vi "Detect Stage Transitions.vi"(1 "Inj Event Boolean State Data":T1) -> (0 "Inj Event Boolean State Data out":T1)   [LabVIEW 2015]
uses:
  Types/Injection Capture Core Boolean State Data.ctl
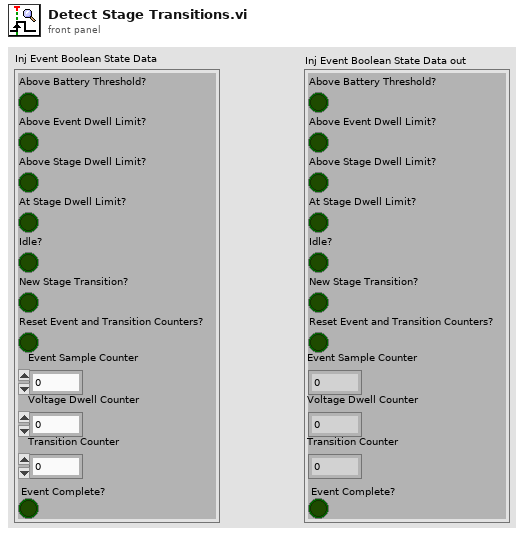
[diagram p1: front panel]
types:
  T1 = typedef "Injection Capture Core Boolean State Data.ctl" = cluster{"Above Battery Threshold?":bool, "Above Event Dwell Limit?":bool, "Above Stage Dwell Limit?":bool, "At Stage Dwell Limit?":bool, "Idle?":bool, "New Stage Transition?":bool, "Reset Event and Transition Counters?":bool, "Event Sample Counter":u16, "Voltage Dwell Counter":u32, "Transition Counter":u8, "Event Complete?":bool}
  T2 = enum8{"Wait for Start", "Wait for Pull-in", "Wait for End"}
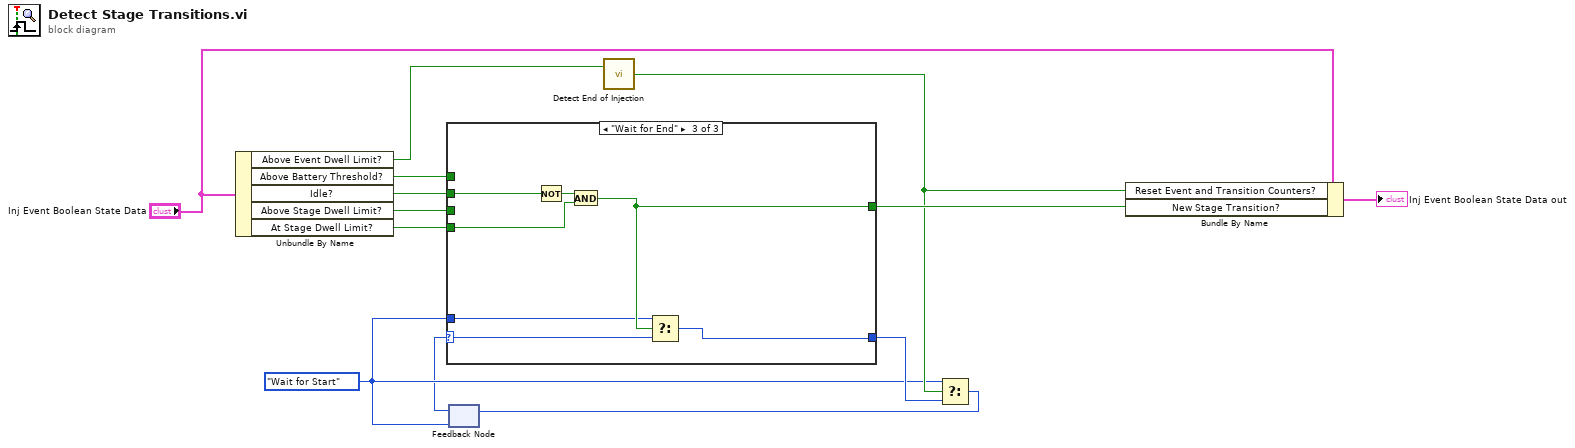
[diagram p0: block diagram]
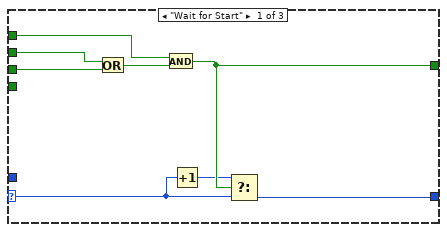
[diagram p2: hidden frame]
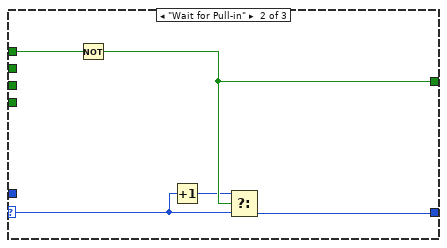
[diagram p3: hidden frame]
diagram:
  w2 = T2."Wait for Start"
  n1 = Unbundle By Name("Inj Event Boolean State Data") -> ("Above Event Dwell Limit?"=w10:bool, "Above Battery Threshold?"=w9:bool, "Idle?"=w11:bool, "Above Stage Dwell Limit?"=w13:bool, "At Stage Dwell Limit?"=w12:bool)
  n2 = feedback #1(w2) -> (w1:T2)
  n3 = case shown="\"Wait for Start\"" w1 {
    selector: w1 -> [w15 w22 w30]
    tunnel: w13 -> [w21 _ _]
    tunnel: w12 -> [_ _ w33]
    tunnel: w11 -> [w20 _ w32]
    tunnel: w9 -> [w18 w25 _]
    tunnel: [w17 w24 w29] -> w7
    tunnel: w2 -> [_ _ w27]
    tunnel: [w14 w26 w28] -> w3
    frame "Wait for Start" {
      n4 = Or(x=w20, y=w21) -> (x .or. y?=w19:bool)
      n5 = And(x=w18, y=w19) -> (x .and. y?=w17:bool)
      n6 = Increment(x=w15) -> (x+1=w16:T2)
      n7 = Select(t=w16, s=w17, f=w15) -> (s? t:f=w14:T2)
    }
    frame "Wait for Pull-in" {
      n8 = Not(x=w25) -> (.not. x?=w24:bool)
      n9 = Increment(x=w22) -> (x+1=w23:T2)
      n10 = Select(t=w23, s=w24, f=w22) -> (s? t:f=w26:T2)
    }
    frame "Wait for End" {
      n11 = Not(x=w32) -> (.not. x?=w31:bool)
      n12 = And(x=w31, y=w33) -> (x .and. y?=w29:bool)
      n13 = Select(t=w27, s=w29, f=w30) -> (s? t:f=w28:T2)
    }
  }
  n14 = call "Detect End of Injection.vi"("Above Event Dwell Limit?"=w10) -> ("Reset Event and Transition Counters?"=w5:bool)  [unwired: 1 in]
  n15 = Select(t=w2, s=w5, f=w3) -> (s? t:f=w4:T2)
  n16 = feedback-in #1(w4) -> ()
  n17 = Bundle By Name(cluster="Inj Event Boolean State Data", "Reset Event and Transition Counters?"=w5, "New Stage Transition?"=w7) -> (→"Inj Event Boolean State Data out":T1)
